vi "UI-产品孔数.vi"(8 "error in (no error)":errorcluster caption="错误输入（无错误）", 11 "名称或相对路径":string="Template Program") -> (0 "error in (no error) 2":errorcluster caption="错误输入（无错误）")   [LabVIEW 2017]
uses:
  Picture/SaveButtom.ctl
  <vilib>/vision/Contour.llb/IMAQ Connect Range Setting.ctl
  <vilib>/vision/Contour.llb/IMAQ Contour Curve Extraction.ctl
  Global System.vi
  <vilib>/Utility/xml.llb/Read From XML File(string).vi
  <vilib>/Utility/xml.llb/Write to XML File(string).vi
panel:
  in  "图像获取":bool
  in  "Curve Extraction (Contour Analysis 1)":T1={"Extraction Mode"=0, "Edge Threshold"=75, "Edge Filter Size"=0, "Min Length"=25, "Search Step Size"=15, "Max Endpoint Gap"=10, "Subpixel"=TRUE} {"Extraction Mode" items=["Normal", "Uniform Regions"]; "Edge Filter Size" items=["Fine", "Normal", "Contour Tracing"]; "Max Endpoint Gap" min=0; "Search Step Size" min=1 max=255 step=1; "Min Length" min=0; "Edge Threshold" min=1 max=350 step=1}
  in  "Match Mode (Contour Analysis 1)":T2
  in  "Template File Path (Contour Analysis 1)":path=path "C:/Users/hedongpo/Desktop/吕亚/Temp3.png"
  in  "Kernel Width (Contour Analysis 1)":u32=5
  in  "Smoothing Kernel (Contour Analysis 1)":u32
  in  "Curve Extraction 2 (Contour Analysis 1)":T1={"Extraction Mode"=0, "Edge Threshold"=75, "Edge Filter Size"=0, "Min Length"=25, "Search Step Size"=15, "Max Endpoint Gap"=10, "Subpixel"=TRUE} {"Extraction Mode" items=["Normal", "Uniform Regions"]; "Edge Filter Size" items=["Fine", "Normal", "Contour Tracing"]; "Max Endpoint Gap" min=0; "Search Step Size" min=1 max=255 step=1; "Min Length" min=0; "Edge Threshold" min=1 max=350 step=1}
  in  "Curve Connection (Contour Analysis 1)":T3[](array[typedef])=[{"Match Constraints"=0, "Min"=1.0, "Max"=12.0}] {"Max" format="%.2f"; "Min" format="%.2f"; "Match Constraints" items=["Distance (pixel)", "Angle Difference (degrees)", "Connectivity Distance (pixel)", "Gradient Difference (degrees)"]}
  in  "Contour Selection (Contour Analysis 1)":T4(ring)
  in  "Search Direction (Contour Analysis 1)":T5(ring)=enum."Annulus Outer To Inner"
  in  "刷新":bool
  in  "测试按钮":bool
  in  "保存按钮":bool
  in  "Main":enum32{"主参数", "显示", "孔数参数设置", "测试效果"}(tab)
  in  "ParamsUI":T6 caption="参数界面" {"Exposure Values" scale=0.0..200000.0}
  out "模板制作":T7(plugin-control)
  in  "抓边参数":T8={"二值化参数"={"Lower value"=104.0, "Upper value"=255.0}, "Selection Values"=[{"Measurement Parameter"=35, "Range Lower Value"=1949.8375244140625, "Range Upper Value"=6069341.0, "Range"=FALSE, "Measurement Type"=FALSE}], "Selection Values2"=[{"Measurement Parameter"=19, "Range Lower Value"=98.74, "Range Upper Value"=135.92, "Range"=FALSE, "Measurement Type"=FALSE}]} caption="参数界面" {"Selection Values2"."Measurement Parameter" items=["Center of Mass X", "Center of Mass Y", "First Pixel X", "First Pixel Y", "Bounding Rect Left", "Bounding Rect Top", "Bounding Rect Right", "Bounding Rect Bottom", "Max Feret Diameter Start X", "Max Feret Diameter Start Y", "Max Feret Diameter End X", "Max Feret Diameter End Y", "Max Horiz. Segment Length Left", "Max Horiz. Segment Length Right", "Max Horiz. Segment Length Row", "-", "Bounding Rect Width", "Bounding Rect Height", "Bounding Rect Diagonal", "Perimeter", "Convex Hull Perimeter", "Holes' Perimeter", "Max Feret Diameter", "Equivalent Ellipse Major Axis", "Equivalent Ellipse Minor Axis", "Equivalent Ellipse Minor Axis (Feret)", "Equivalent Rect Long Side", "Equivalent Rect Short Side", "Equivalent Rect Diagonal", "Equivalent Rect Short Side (Feret)", "Average Horiz. Segment Length", "Average Vert. Segment Length", "Hydraulic Radius", "Waddel Disk Diameter", "-", "Area", "Holes' Area", "Particle & Holes' Area", "Convex Hull Area", "Image Area", "-", "Number of Holes", "Number of Horiz. Segments", "Number of Vert. Segments", "-", "Orientation", "Max Feret Diameter Orientation", "-", "% Area/Image Area", "% Area/(Particle & Holes' Area)", "Ratio of Equivalent Ellipse Axes", "Ratio of Equivalent Rect Sides", "-", "Elongation Factor", "Compactness Factor", "Heywood Circularity Factor", "Type Factor", "-", "Sum X", "Sum Y", "Sum XX", "Sum XY", "Sum YY", "Sum XXX", "Sum XXY", "Sum XYY", "Sum YYY", "-", "Moment of Inertia XX", "Moment of Inertia XY", "Moment of Inertia YY", "Moment of Inertia XXX", "Moment of Inertia XXY", "Moment of Inertia XYY", "Moment of Inertia YYY", "Norm. Moment of Inertia XX", "Norm. Moment of Inertia XY", "Norm. Moment of Inertia YY", "Norm. Moment of Inertia XXX", "Norm. Moment of Inertia XXY", "Norm. Moment of Inertia XYY", "Norm. Moment of Inertia YYY", "Hu Moment 1", "Hu Moment 2", "Hu Moment 3", "Hu Moment 4", "Hu Moment 5", "Hu Moment 6", "Hu Moment 7"]; "Selection Values"."Measurement Parameter" items=["Center of Mass X", "Center of Mass Y", "First Pixel X", "First Pixel Y", "Bounding Rect Left", "Bounding Rect Top", "Bounding Rect Right", "Bounding Rect Bottom", "Max Feret Diameter Start X", "Max Feret Diameter Start Y", "Max Feret Diameter End X", "Max Feret Diameter End Y", "Max Horiz. Segment Length Left", "Max Horiz. Segment Length Right", "Max Horiz. Segment Length Row", "-", "Bounding Rect Width", "Bounding Rect Height", "Bounding Rect Diagonal", "Perimeter", "Convex Hull Perimeter", "Holes' Perimeter", "Max Feret Diameter", "Equivalent Ellipse Major Axis", "Equivalent Ellipse Minor Axis", "Equivalent Ellipse Minor Axis (Feret)", "Equivalent Rect Long Side", "Equivalent Rect Short Side", "Equivalent Rect Diagonal", "Equivalent Rect Short Side (Feret)", "Average Horiz. Segment Length", "Average Vert. Segment Length", "Hydraulic Radius", "Waddel Disk Diameter", "-", "Area", "Holes' Area", "Particle & Holes' Area", "Convex Hull Area", "Image Area", "-", "Number of Holes", "Number of Horiz. Segments", "Number of Vert. Segments", "-", "Orientation", "Max Feret Diameter Orientation", "-", "% Area/Image Area", "% Area/(Particle & Holes' Area)", "Ratio of Equivalent Ellipse Axes", "Ratio of Equivalent Rect Sides", "-", "Elongation Factor", "Compactness Factor", "Heywood Circularity Factor", "Type Factor", "-", "Sum X", "Sum Y", "Sum XX", "Sum XY", "Sum YY", "Sum XXX", "Sum XXY", "Sum XYY", "Sum YYY", "-", "Moment of Inertia XX", "Moment of Inertia XY", "Moment of Inertia YY", "Moment of Inertia XXX", "Moment of Inertia XXY", "Moment of Inertia XYY", "Moment of Inertia YYY", "Norm. Moment of Inertia XX", "Norm. Moment of Inertia XY", "Norm. Moment of Inertia YY", "Norm. Moment of Inertia XXX", "Norm. Moment of Inertia XXY", "Norm. Moment of Inertia XYY", "Norm. Moment of Inertia YYY", "Hu Moment 1", "Hu Moment 2", "Hu Moment 3", "Hu Moment 4", "Hu Moment 5", "Hu Moment 6", "Hu Moment 7"]; "Selection Values"."Range Upper Value" format="%#_9f"}
  in  "测试结果":string[][](table)=[["", ""]]
  out "原始图像":T7(plugin-control)
  out "处理后图像":T7(plugin-control)
  out "路径输出":path
  out "添加的路径":path
  in  "Vision Paramter Save Buttom":T9
  out "system time":string
  in  "取消按钮":bool
  # "Range"
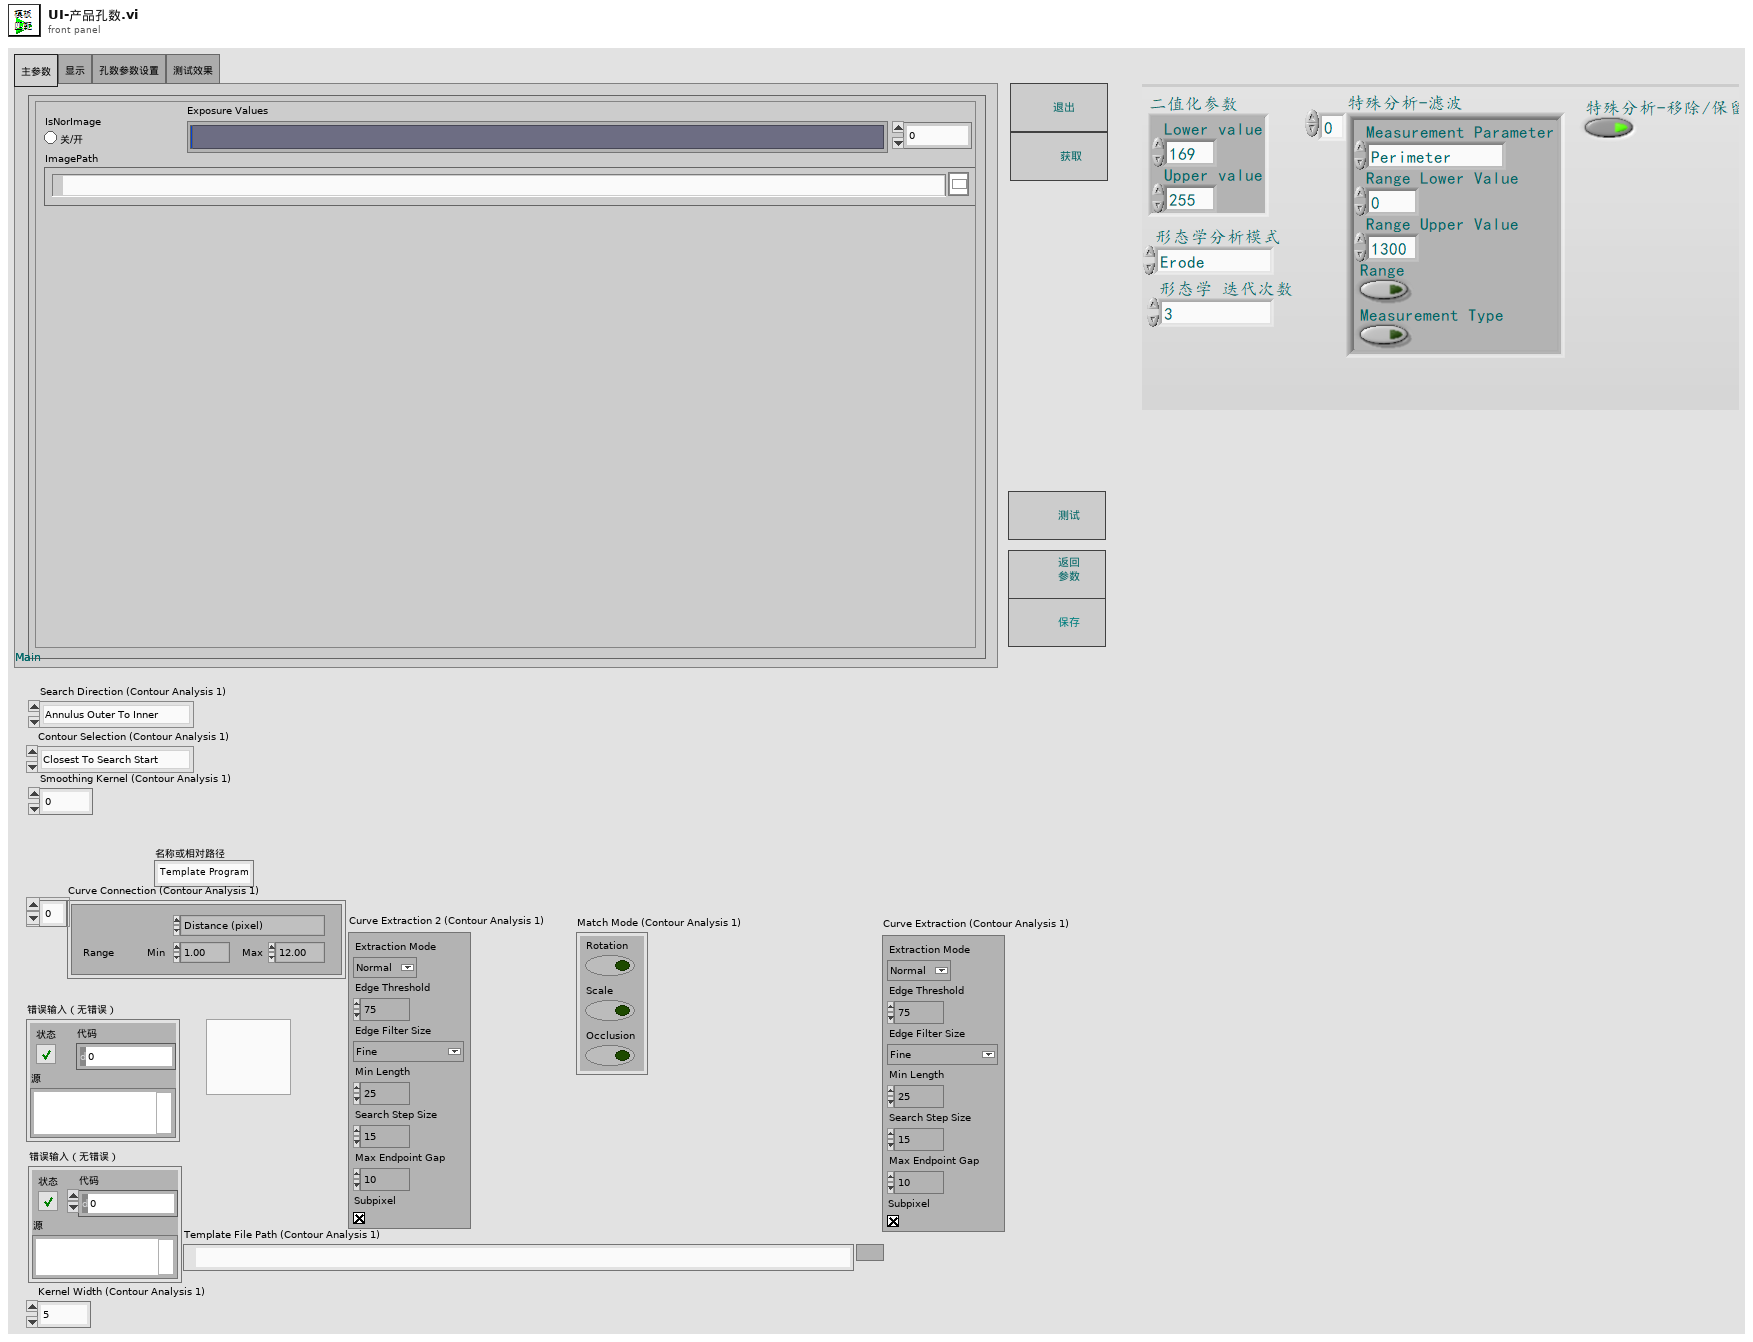
[diagram p1: front panel]
types:
  T1 = typedef "IMAQ Contour Curve Extraction.ctl" = cluster{"Extraction Mode":u32, "Edge Threshold":i32, "Edge Filter Size":u32, "Min Length":i32, "Search Step Size":i32, "Max Endpoint Gap":i32, "Subpixel":bool}
  T2 = cluster{"Rotation":bool, "Scale":bool, "Occlusion":bool}
  T3 = typedef "IMAQ Connect Range Setting.ctl" = cluster{"Match Constraints":u32, "Min":dbl, "Max":dbl}
  T4 = enum16{"Closest To Search Start", "Maximum Length", "Strongest Mean Gradient Change"}
  T5 = enum16{"Rect Left To Right", "Rect Right To Left", "Rect Top To Bottom", "Rect Bottom To Top", "Annulus Inner To Outer", "Annulus Outer To Inner", "Annulus Start Angle To End Angle", "Annulus End Angle To Start Angle"}
  T6 = cluster{"IsNorImage":bool, "Exposure Values":u32, "ImagePath":path}
  T7 = typedef "IMAQ Image.ctl" = refnum<image>
  T8 = cluster{"二值化参数":cluster{"Lower value":sgl, "Upper value":sgl}, "Selection Values":cluster{"Measurement Parameter":i32, "Range Lower Value":dbl, "Range Upper Value":dbl, "Range":bool, "Measurement Type":bool}[], "Selection Values2":cluster{"Measurement Parameter":i32, "Range Lower Value":dbl, "Range Upper Value":dbl, "Range":bool, "Measurement Type":bool}[]}
  T9 = typedef "SaveButtom.ctl" = bool
  T10 = cluster{"index":i32, "this vi":refnum<vi>, "error out":errorcluster}
  T11 = cluster{"master data":string, "priority":u16, "secondary data":string[]}
  T12 = cluster{"case name":string[], "queue array":refnum<queue>[]}
  T13 = typedef "Image Type" = u32
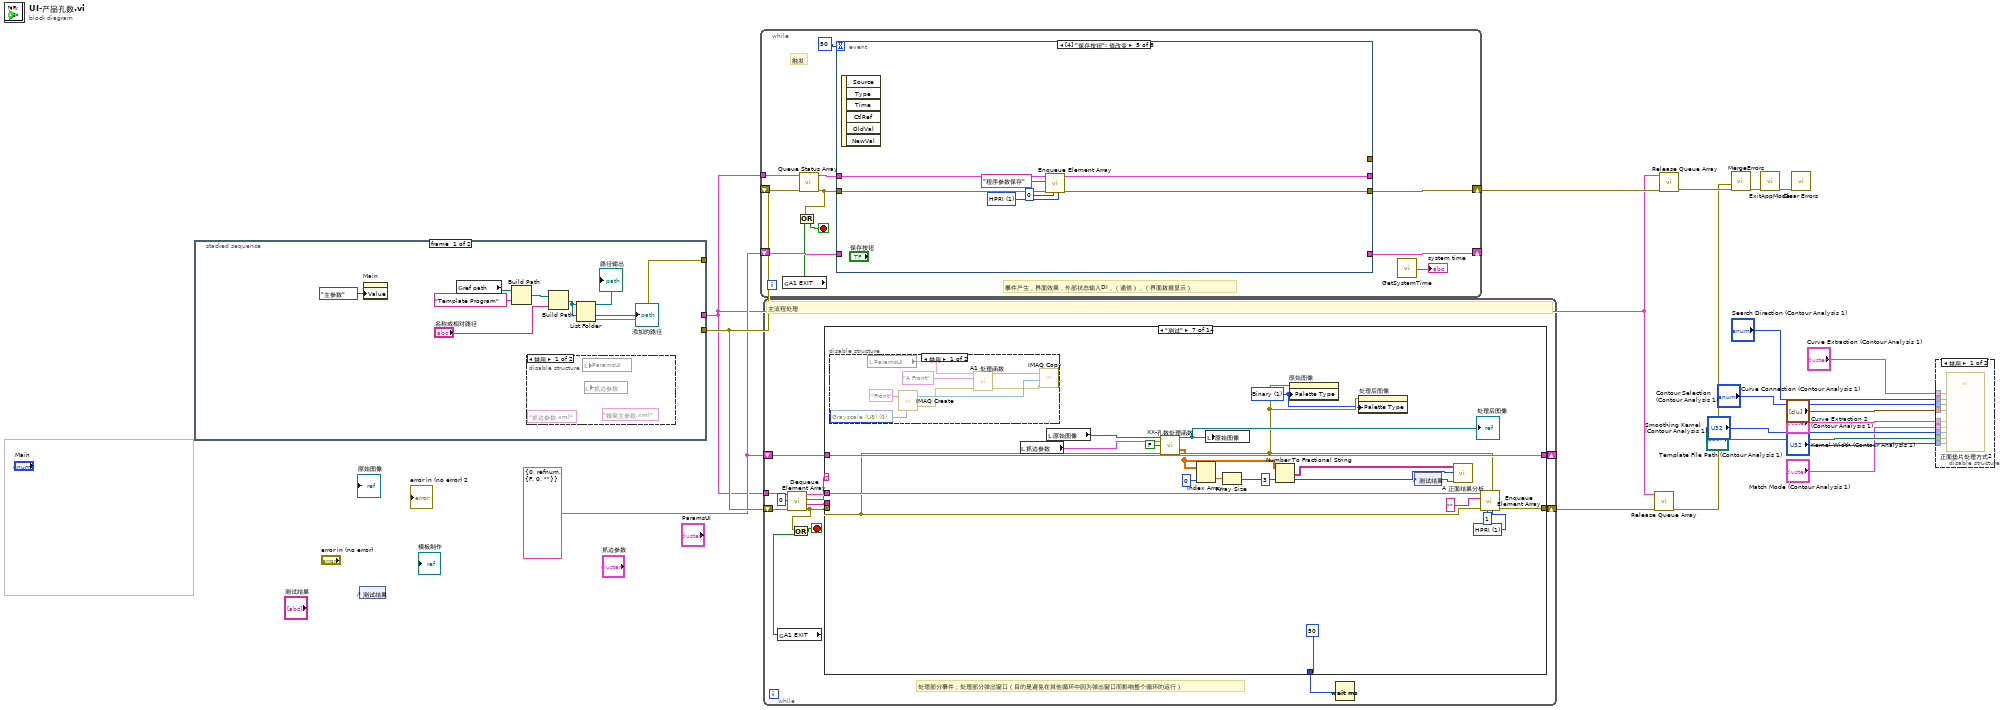
[diagram p0: block diagram]
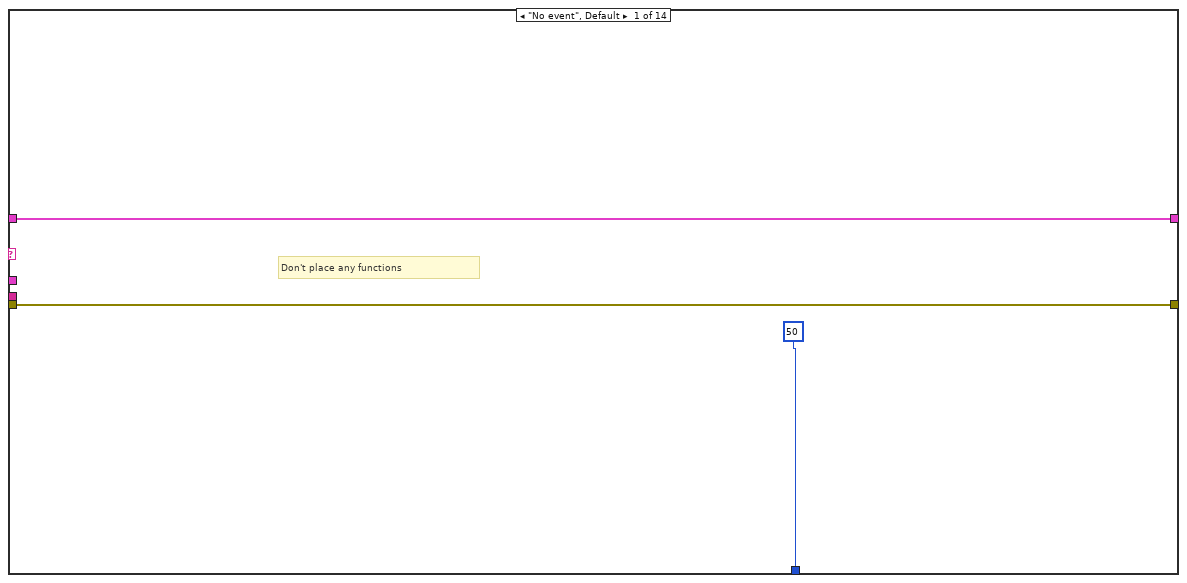
[diagram p3: hidden frame]
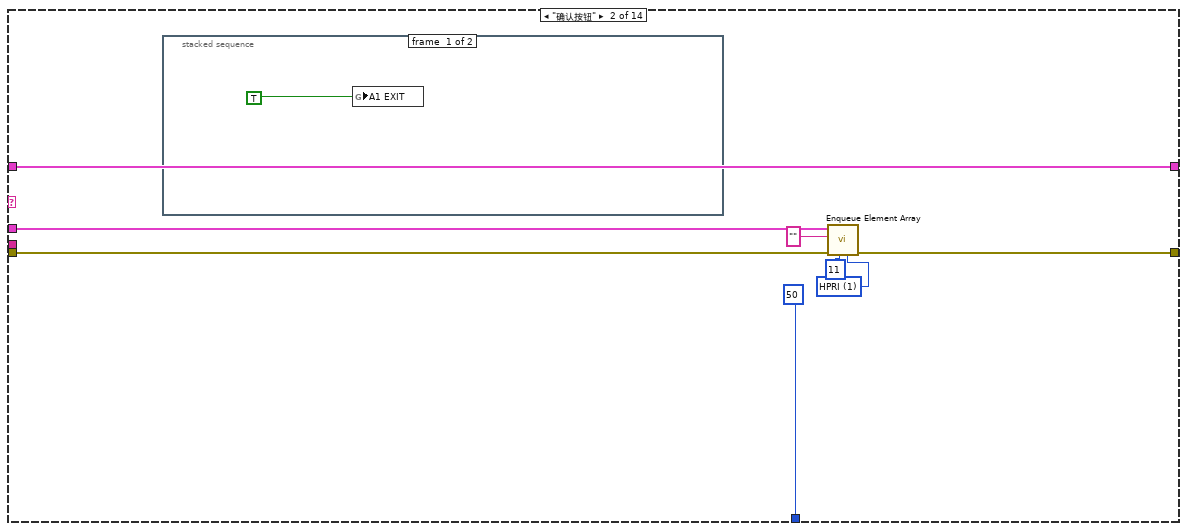
[diagram p4: hidden frame]
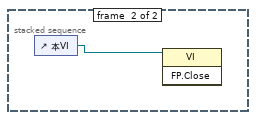
[diagram p5: hidden frame]
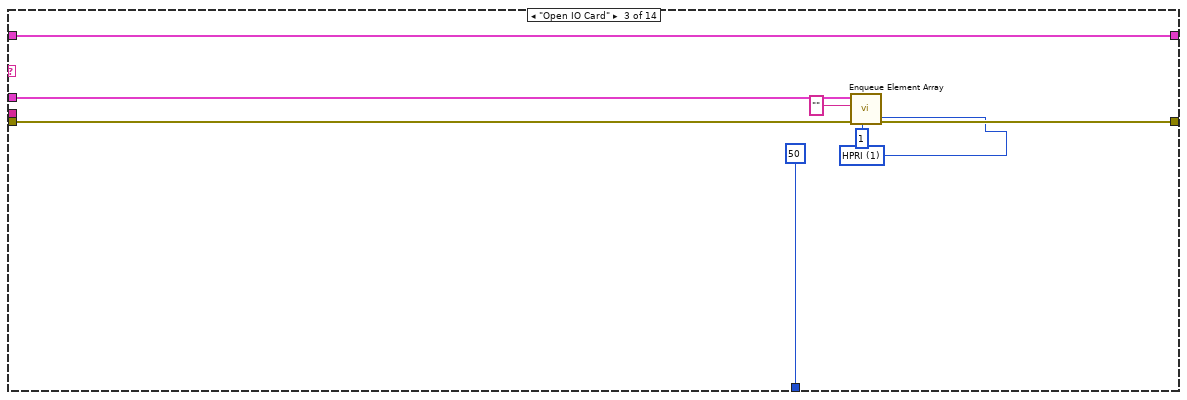
[diagram p6: hidden frame]
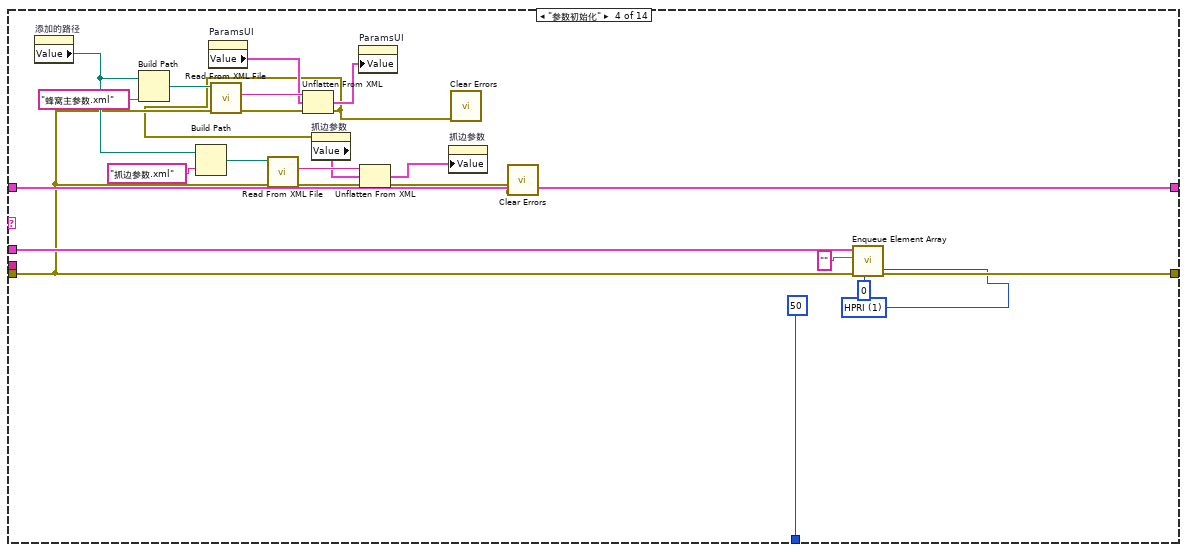
[diagram p7: hidden frame]
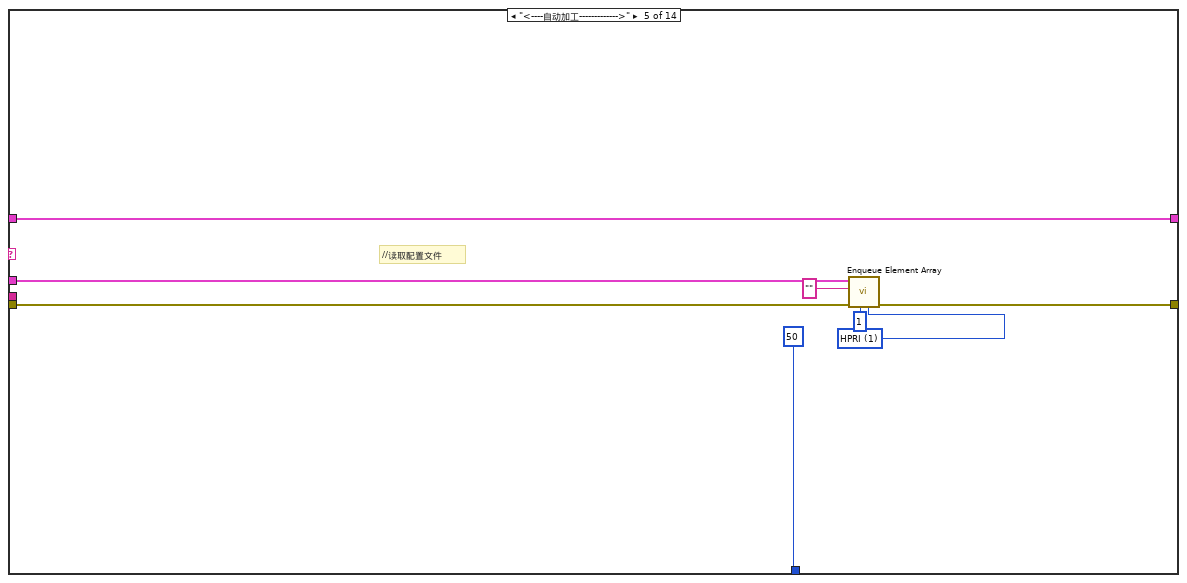
[diagram p8: hidden frame]
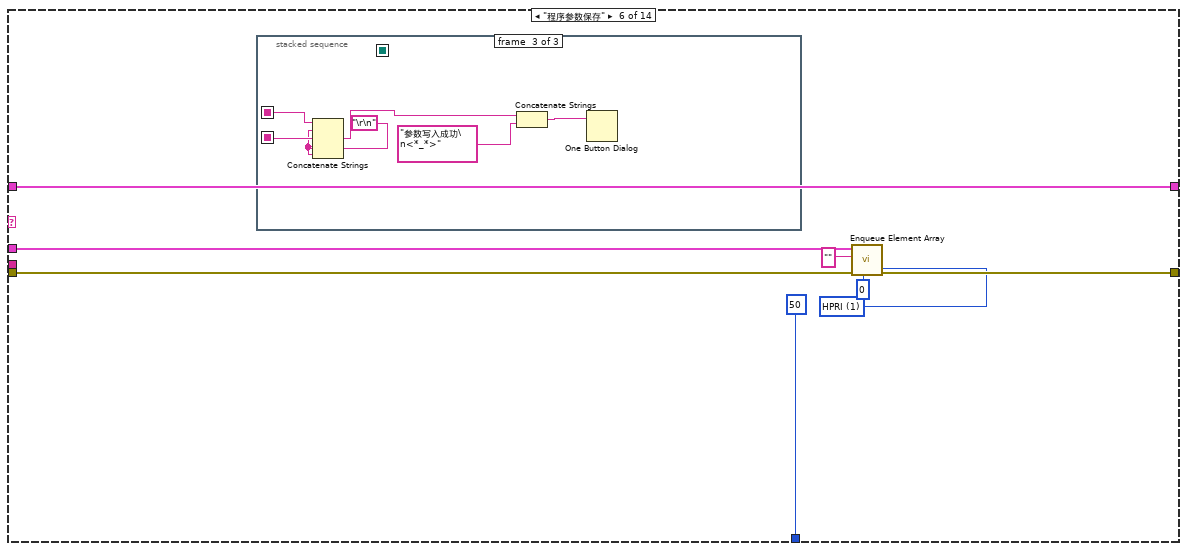
[diagram p9: hidden frame]
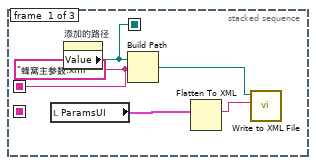
[diagram p10: hidden frame]
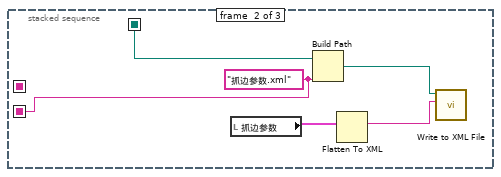
[diagram p11: hidden frame]
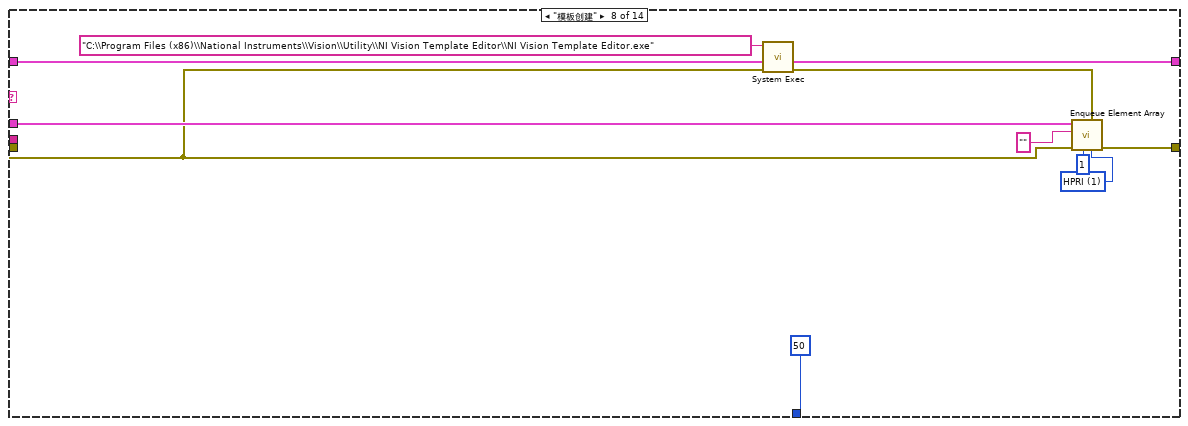
[diagram p13: hidden frame]
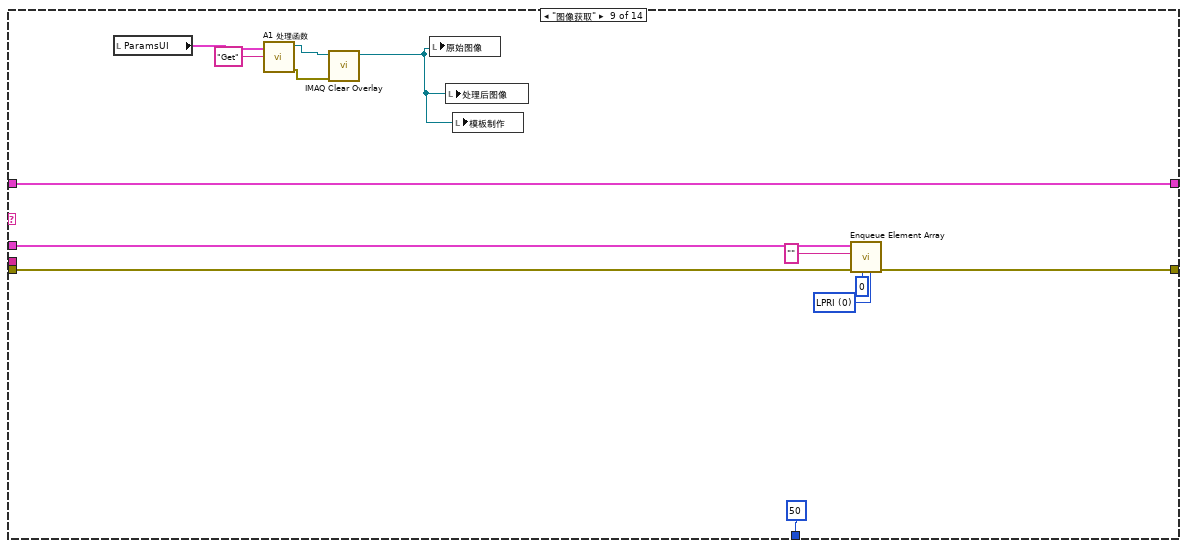
[diagram p14: hidden frame]
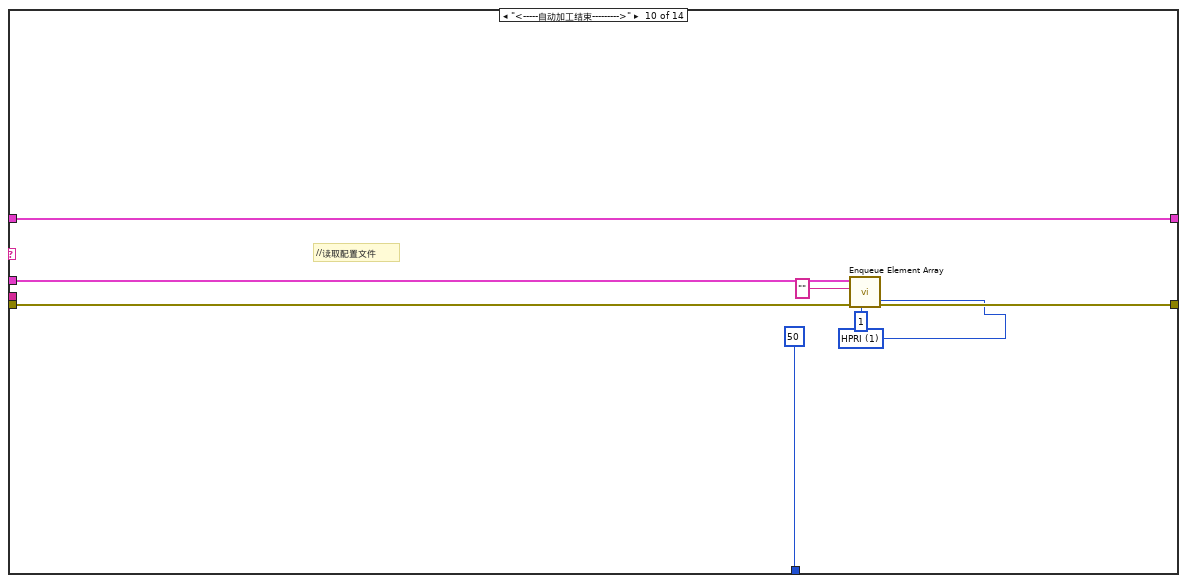
[diagram p15: hidden frame]
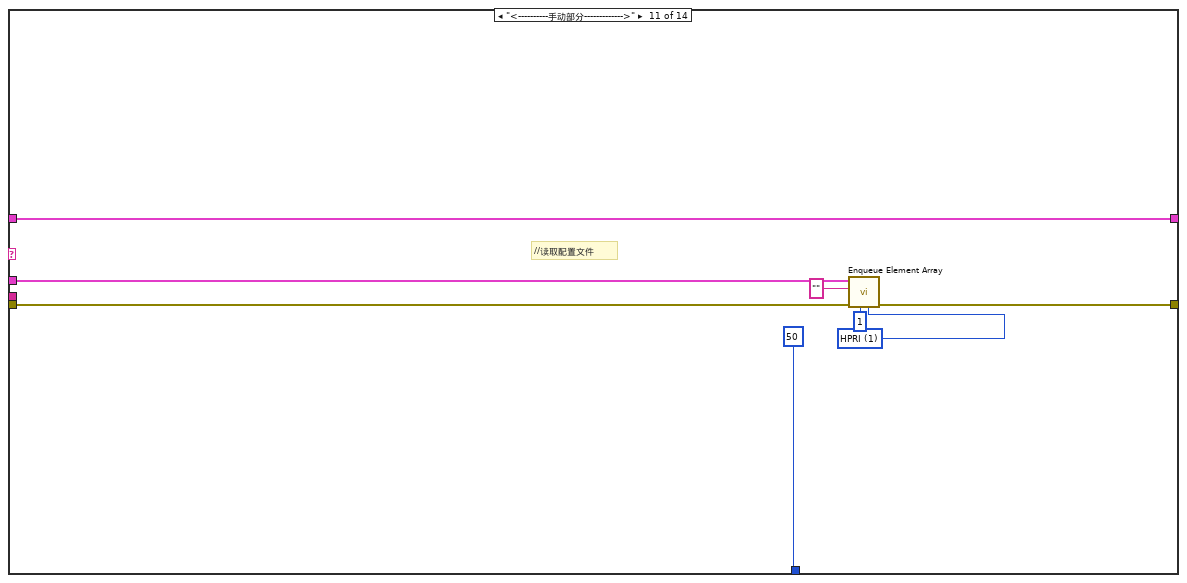
[diagram p16: hidden frame]
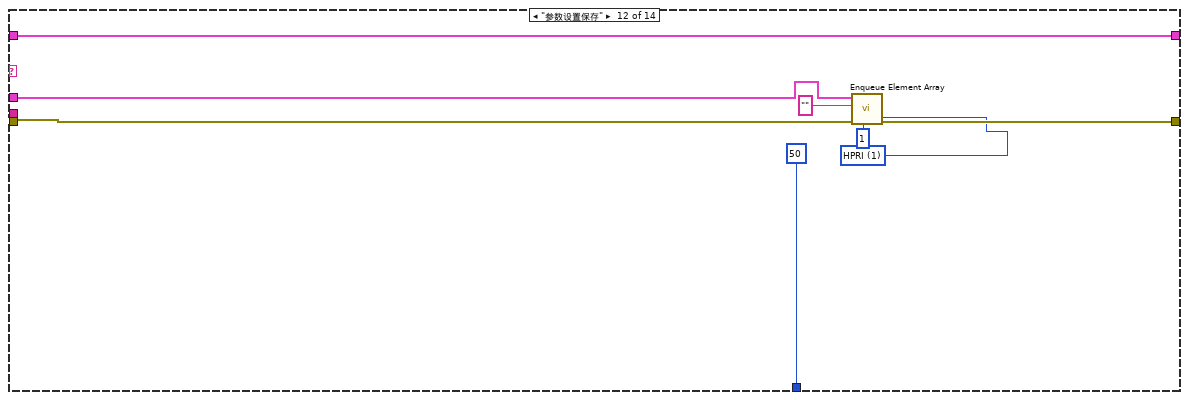
[diagram p17: hidden frame]
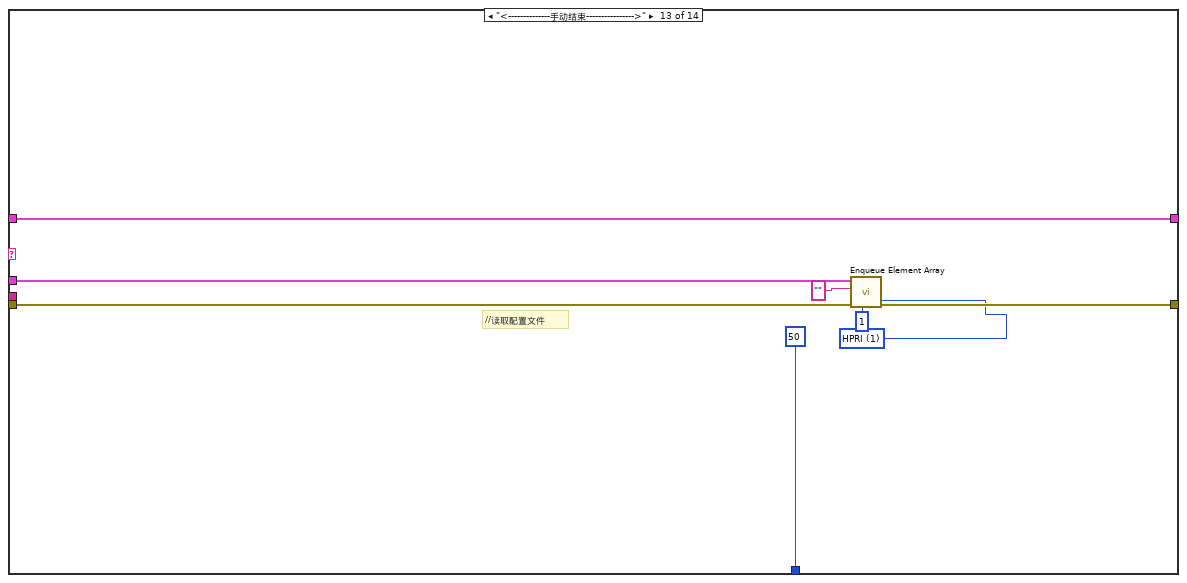
[diagram p18: hidden frame]
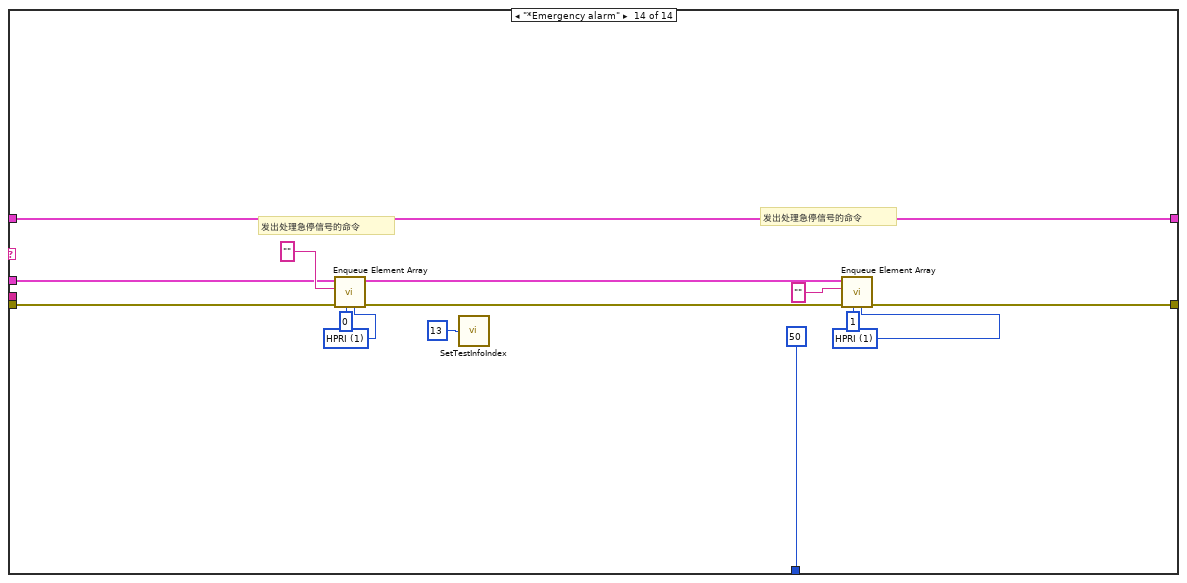
[diagram p19: hidden frame]
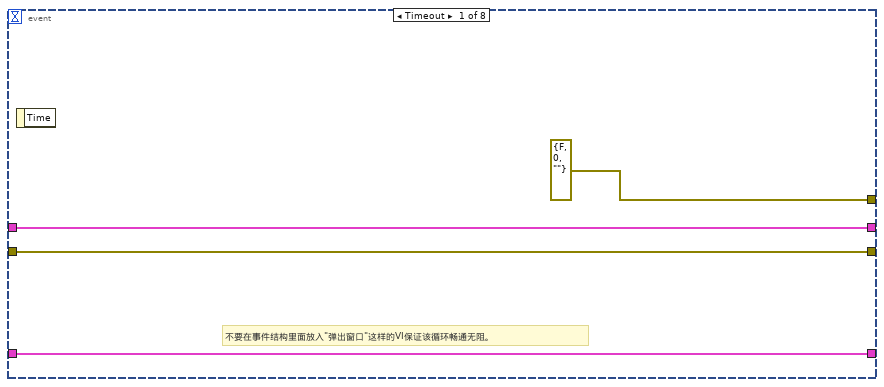
[diagram p20: hidden frame]
diagram:
  w13 = T10 {"index"=0, "this vi"=refnum, "error out"={"status"=FALSE, "code"=0, "source"=""}} ("parameter buffer")
  n1 = stacked-sequence {
    tunnel: [w24 _] -> _
    tunnel: [_ w28] -> w14
    tunnel: [_ w27] -> w10
    frame #0 {
      n2 = property on="Main" class="TabCtl (严格)"("Value"=enum32{"主参数", "显示", "孔数参数设置", "测试效果"}."主参数" ("Main")) -> ()  [unwired: 2 in, 2 out]
      n3 = global read "Global System.vi" "ref path"() -> (w22:path)
      n4 = Build Path(base path=w22, name or relative path="Template Program" ("名称或相对路径")) -> (appended path=w20:path)
      n5 = disable-structure shown="禁用" {
        frame Disabled {
          (unwired) "抓边参数.xml" ("名称或相对路径")
          (unwired) "蜂窝主参数.xml" ("名称或相对路径")
          n6 = local read "ParamsUI"() -> ()  [unwired: 1 in]
          n7 = local read "抓边参数"() -> ()  [unwired: 1 in]
        }
        frame Enabled {
        }
      }
      n8 = Build Path(base path=w20, name or relative path="名称或相对路径") -> (appended path=w26:path)
      "添加的路径" <- w26
      n9 = List Folder(path=w26) -> (path out=→"路径输出":path, error out=w24:errorcluster)  [unwired: 3 in, 2 out]
    }
    frame #1 {
      w36 = string[] ["comm queue1", "data queue 11", "data queue 12", "data queue 13", "data queue 14"]  # queue name
      w37 = 4  # queue num
      w38 = T11 {"master data"="", "priority"=0, "secondary data"=[]}  # element data type
      n10 = call "Obtain Queue Array.vi"("queue name"=w36, "element data type"=w38, "queue num"=w37) -> ("error out"=w32:errorcluster, "queue out"=w33:T12)  [unwired: 2 in, 1 out]
      n11 = call "Enqueue Element Array.vi"("queue index"=0, "error in"=w32, "master data"="参数初始化", "queue in"=w33) -> ("error out"=w31:errorcluster, "queue out"=w30:T12)  [unwired: 6 in]
      n12 = disable-structure shown="启用" {
        disable-tunnel: w31 -> [w44 w45]
        disable-tunnel: w30 -> [w43 w46]
        disable-tunnel: "Loading Variable" ("master data") -> [w42 _]
        disable-tunnel: [w40 w45] -> w28
        disable-tunnel: [w39 w46] -> w27
        frame Disabled {
          n13 = call "Enqueue Element Array.vi"("queue index"=12, "error in"=w44, "master data"=w42, "queue in"=w43) -> ("error out"=w40:errorcluster, "queue out"=w39:T12)  [unwired: 6 in]
        }
        frame Enabled {
        }
      }
    }
  }
  n14 = control-ref of="测试结果"() -> ()  [unwired: 1 out]
  n15 = while {
    shift-right: [w50] -> w15
    shift-left: w14 -> [w54]
    shift-right: [w52] -> _
    shift-left: w13 -> [w53]
    tunnel: w10 -> [w56]
    stop <- w47 stop-if-true
    # "触发"
    # "事件产生，界面效果，外部状态输入DI，（通信），（界面数据显示）"
    n16 = global read "Global System.vi" "A1 EXIT"() -> (w48:bool)
    n17 = call "Queue Status Array.vi"("error in (no error)"=w54, "queue in"=w56) -> ("error out"=w49:errorcluster, "queue out"=w51:T12)  [unwired: 4 in]
    n18 = Or(x=w49, y=w48) -> (x .or. y?=w47:bool)
    n19 = event shown="[4] \"保存按钮\": 值改变" {
      selector: _ -> [_ _ _ _ _ _ _ _]
      dyn-events: _ -> [_ _ _ _ _ _ _ _]
      timeout: 50 -> [_ _ _ _ _ _ _ _]
      tunnel: w53 -> [w61 w69 _ _ _ _ _ _]
      tunnel: [w61 w69 _ _ _ _ _ _] -> w52
      tunnel: [errorcluster {"status"=FALSE, "code"=0, "source"=""} ("error out") _ _ _ _ _ _ _] -> _
      tunnel: w51 -> [w59 w68 w74 w81 w88 w96 w104 w112]
      tunnel: w49 -> [w58 w67 w73 w80 w87 w95 w103 w111]
      tunnel: [w58 w66 w71 w78 w85 w93 w101 w109] -> w50
      tunnel: [w59 w65 w72 w79 w86 w94 w102 w110] -> _
      event Timeout {
        # "不要在事件结构里面放入\"弹出窗口\"这样的VI保证该循环畅通无阻。"
        n20 = event-data() -> ()  [unwired: 1 in, 1 out]
      }
      event Panel Close? {
        w63 = u16 1 items=["HPRI"=1, "LPRI"=0] ("priority")
        n21 = event-data() -> ()  [unwired: 1 in, 4 out]
        n22 = call "Enqueue Element Array.vi"("priority"=w63, "queue index"=0, "error in"=w67, "master data"="*Exit application", "queue in"=w68) -> ("error out"=w66:errorcluster, "queue out"=w65:T12)  [unwired: 5 in]
        n23 = event-data("Discard?"=TRUE) -> ()  [unwired: 1 in, 1 out]
      }
      event Value Change {
        w76 = u16 1 items=["HPRI"=1, "LPRI"=0] ("priority")
        n24 = event-data() -> ()  [unwired: 1 in, 6 out]
        n25 = call "Enqueue Element Array.vi"("priority"=w76, "queue index"=0, "error in"=w73, "master data"="Vision Paramter Save", "queue in"=w74) -> ("error out"=w71:errorcluster, "queue out"=w72:T12)  [unwired: 5 in]
      }
      event "取消按钮": Value Change {
        w83 = u16 1 items=["HPRI"=1, "LPRI"=0] ("priority")
        n26 = event-data() -> ()  [unwired: 1 in, 6 out]
        n27 = call "Enqueue Element Array.vi"("priority"=w83, "queue index"=0, "error in"=w80, "master data"="确认按钮", "queue in"=w81) -> ("error out"=w78:errorcluster, "queue out"=w79:T12)  [unwired: 5 in]
      }
      event "保存按钮": Value Change {
        w90 = u16 1 items=["HPRI"=1, "LPRI"=0] ("priority")
        n28 = event-data() -> ()  [unwired: 1 in, 6 out]
        n29 = call "Enqueue Element Array.vi"("priority"=w90, "queue index"=0, "error in"=w87, "master data"="程序参数保存", "queue in"=w88) -> ("error out"=w85:errorcluster, "queue out"=w86:T12)  [unwired: 5 in]
      }
      event "测试按钮": Value Change {
        (unwired) "模板匹配抓边测试"
        w98 = u16 1 items=["HPRI"=1, "LPRI"=0] ("priority")
        n30 = event-data() -> ()  [unwired: 1 in, 6 out]
        n31 = property on="Main" class="TabCtl (严格)"("Value"=enum32{"主参数", "显示", "孔数参数设置", "测试效果"}."测试效果" ("Main")) -> ()  [unwired: 2 in, 2 out]
        n32 = call "Enqueue Element Array.vi"("priority"=w98, "queue index"=0, "error in"=w95, "master data"="测试", "queue in"=w96) -> ("error out"=w93:errorcluster, "queue out"=w94:T12)  [unwired: 5 in]
      }
      event "图像获取": Value Change {
        w106 = u16 1 items=["HPRI"=1, "LPRI"=0] ("priority")
        n33 = event-data() -> ()  [unwired: 1 in, 6 out]
        n34 = property on="Main" class="TabCtl (严格)"("Value"=enum32{"主参数", "显示", "孔数参数设置", "测试效果"}."显示" ("Main")) -> ()  [unwired: 2 in, 2 out]
        n35 = call "Enqueue Element Array.vi"("priority"=w106, "queue index"=0, "error in"=w103, "master data"="图像获取", "queue in"=w104) -> ("error out"=w101:errorcluster, "queue out"=w102:T12)  [unwired: 5 in]
      }
      event "刷新": Value Change {
        n36 = event-data() -> ()  [unwired: 1 in, 6 out]
        n37 = disable-structure shown="禁用" {
          disable-tunnel: w112 -> [w116 _]
          disable-tunnel: w111 -> [w115 _]
          disable-tunnel: [w114 _] -> w110
          disable-tunnel: [w113 _] -> w109
          frame Disabled {
            w118 = u16 1 items=["HPRI"=1, "LPRI"=0] ("priority")
            # "刷新"
            n38 = call "Enqueue Element Array.vi"("priority"=w118, "queue index"=0, "error in"=w115, "master data"="刷新", "queue in"=w116) -> ("error out"=w113:errorcluster, "queue out"=w114:T12)  [unwired: 5 in]
          }
          frame Enabled {
          }
        }
        n39 = property on="Main" class="TabCtl (严格)"("Value"=enum32{"主参数", "显示", "孔数参数设置", "测试效果"}."主参数" ("Main")) -> ()  [unwired: 2 in, 2 out]
      }
    }
    n40 = call "GetSystemTime.vi"() -> ("date/time string"=→"system time":string)  [unwired: 7 in]
  }
  n41 = while {
    shift-right: [w132] -> w12
    shift-left: w14 -> [w123]
    shift-right: [w129] -> _
    shift-left: w13 -> [w130]
    tunnel: w10 -> [w125]
    stop <- w120 stop-if-true
    # "处理部分事件；处理部分弹出窗口（目的是避免在其他循环中因为弹出窗口而影响整个循环的运行）"
    # "主流程处理"
    n42 = global read "Global System.vi" "A1 EXIT"() -> (w121:bool)
    n43 = call "Dequeue Element Array.vi"("queue in"=w125, "queue index"=0, "error in"=w123) -> ("queue out"=w128:T12, "master data"=w127:string, "secondary data"=w126:string[], "error out"=w122:errorcluster)  [unwired: 2 in, 1 out]
    n44 = Or(x=w122, y=w121) -> (x .or. y?=w120:bool)
    n45 = case shown="\"测试\"" w127 {
      tunnel: w128 -> [_ w142 w152 w175 w183 w185 w228 w246 w259 w267 w275 w283 w291 w297]
      tunnel: w122 -> [w134 w138 w148 w157 w179 w189 w219 w240 w253 w263 w271 w279 w287 w294]
      tunnel: [w134 w141 w151 w174 w182 w191 w227 w245 w258 w266 w274 w282 w290 w305] -> w132
      tunnel: [50 50 50 50 50 50 50 50 50 50 50 50 50 50] -> w131
      tunnel: w130 -> [w135 w139 w149 w170 w180 w186 w226 w241 w254 w264 w272 w280 w288 w303]
      tunnel: [w135 w139 w149 w170 w180 w186 w226 w241 w254 w264 w272 w280 w288 w303] -> w129
      tunnel: w126 -> [_ _ _ _ _ _ _ _ _ _ _ _ _ _]
      frame "No event", Default {
        # "Don't place any functions"
      }
      frame "确认按钮" {
        w136 = u16 1 items=["HPRI"=1, "LPRI"=0] ("priority")
        n46 = stacked-sequence {
          frame #0 {
            n47 = global write "Global System.vi" "A1 EXIT"(TRUE ("EXIT")) -> ()
          }
          frame #1 {
            n48 = control-ref of="本VI"() -> (w145:refnum<vi>)
            n49 = invoke class="VI" method="FP.Close"(reference=w145) -> ()  [unwired: 2 in, 3 out]
          }
        }
        n50 = call "Enqueue Element Array.vi"("priority"=w136, "queue index"=11, "error in"=w138, "master data"="" ("Element 1"), "queue in"=w142) -> ("error out"=w141:errorcluster)  [unwired: 5 in, 1 out]
      }
      frame "Open IO Card" {
        w146 = u16 1 items=["HPRI"=1, "LPRI"=0] ("priority")
        n51 = call "Enqueue Element Array.vi"("priority"=w146, "queue index"=1, "error in"=w148, "master data"="" ("Element 1"), "queue in"=w152) -> ("error out"=w151:errorcluster)  [unwired: 5 in, 1 out]
      }
      frame "参数初始化" {
        w171 = u16 1 items=["HPRI"=1, "LPRI"=0] ("priority")
        n52 = property on="添加的路径" class="Path"() -> ("Value"=w159:path)  [unwired: 2 in, 2 out]
        n53 = Build Path(base path=w159, name or relative path="蜂窝主参数.xml" ("名称或相对路径")) -> (appended path=w168:path)
        n54 = Build Path(base path=w159, name or relative path="抓边参数.xml" ("名称或相对路径")) -> (appended path=w160:path)
        n55 = property on="ParamsUI" class="Clust (严格)"() -> ("Value"=w166:T6)  [unwired: 2 in, 2 out]
        n56 = call-poly <vilib>:"Read From XML File.vi"("error in (no error)"=w157, "XML File Path"=w168) -> ("error out"=w164:errorcluster, "XML Elements"=w167:string)  [unwired: 7 in, 1 out]
        n57 = call-poly <vilib>:"Read From XML File.vi"("error in (no error)"=w157, "XML File Path"=w160) -> ("error out"=w162:errorcluster, "XML Elements"=w161:string)  [unwired: 7 in, 1 out]
        n58 = Unflatten From XML(xml string=w167, type=w166, error in (no error)=w164) -> (value=w165:T6, error out=w156:errorcluster)
        n59 = property on="抓边参数" class="Clust (严格)"(error in=w156) -> ("Value"=w155:T8)  [unwired: 1 in, 2 out]
        n60 = property on="ParamsUI" class="Clust (严格)"("Value"=w165) -> ()  [unwired: 2 in, 2 out]
        n61 = Unflatten From XML(xml string=w161, type=w155, error in (no error)=w162) -> (value=w154:T8, error out=w163:errorcluster)
        n62 = property on="抓边参数" class="Clust (严格)"("Value"=w154) -> ()  [unwired: 2 in, 2 out]
        n63 = call <vilib>:"Clear Errors.vi"("error in (no error)"=w156) -> ()  [unwired: 5 in, 2 out]
        n64 = call <vilib>:"Clear Errors.vi"("error in (no error)"=w163) -> ()  [unwired: 5 in, 2 out]
        n65 = call "Enqueue Element Array.vi"("priority"=w171, "queue index"=0, "error in"=w157, "master data"="" ("Element 1"), "queue in"=w175) -> ("error out"=w174:errorcluster)  [unwired: 5 in, 1 out]
      }
      frame "<----自动加工------------->" {
        w177 = u16 1 items=["HPRI"=1, "LPRI"=0] ("priority")
        # "//读取配置文件"
        n66 = call "Enqueue Element Array.vi"("priority"=w177, "queue index"=1, "error in"=w179, "master data"="" ("Element 1"), "queue in"=w183) -> ("error out"=w182:errorcluster)  [unwired: 5 in, 1 out]
      }
      frame "程序参数保存" {
        w187 = u16 1 items=["HPRI"=1, "LPRI"=0] ("priority")
        n67 = stacked-sequence {
          seq-local: [w195 _ _] -> [_ _ w206]
          seq-local: [_ w201 _] -> [_ _ w205]
          seq-local: [w194 _ _] -> [_ w200 _]
          frame #0 {
            w195 = "蜂窝主参数.xml" ("名称或相对路径")
            n68 = local read "ParamsUI"() -> (w193:T6)
            n69 = property on="添加的路径" class="Path"() -> ("Value"=w194:path)  [unwired: 2 in, 2 out]
            n70 = Build Path(base path=w194, name or relative path=w195) -> (appended path=w196:path)
            n71 = Flatten To XML(anything=w193) -> (xml string=w197:string)
            n72 = call-poly <vilib>:"Write to XML File.vi"("XML Input"=w197, "XML File Path"=w196) -> ()  [unwired: 7 in, 3 out]
          }
          frame #1 {
            w201 = "抓边参数.xml" ("名称或相对路径")
            n73 = local read "抓边参数"() -> (w198:T8)
            n74 = Build Path(base path=w200, name or relative path=w201) -> (appended path=w202:path)
            n75 = Flatten To XML(anything=w198) -> (xml string=w199:string)
            n76 = call-poly <vilib>:"Write to XML File.vi"("XML Input"=w199, "XML File Path"=w202) -> ()  [unwired: 7 in, 3 out]
          }
          frame #2 {
            w203 = "\r\n"
            n77 = Concatenate Strings(w206, w203, w205, w203, w203) -> (w204:string)
            n78 = Concatenate Strings(w204, "参数写入成功\n<*_*>" ("消息")) -> (w207:string)
            n79 = One Button Dialog(message=w207) -> ()  [unwired: 1 in, 1 out]
          }
        }
        n80 = call "Enqueue Element Array.vi"("priority"=w187, "queue index"=0, "error in"=w189, "master data"="" ("Element 1"), "queue in"=w185) -> ("error out"=w191:errorcluster)  [unwired: 5 in, 1 out]
      }
      frame "测试" {
        w215 = u32 1 items=["Grayscale", "Binary", "Gradient", "Rainbow", "Temperature", "User Defined", "Binary 16 Bit", "Gradient 16 Bit", "Rainbow 16 Bit", "Temperature 16 Bit", "User Defined 16 Bit"] ("Palette:Palette Type")
        w223 = u16 1 items=["HPRI"=1, "LPRI"=0] ("priority")
        n81 = disable-structure shown="禁用" {
          frame Disabled {
            w236 = T13 0 items=["Grayscale (U8)", "Grayscale (I16)", "Grayscale (SGL)", "Complex (CSG)", "RGB (U32)", "HSL (U32)", "RGB (U64)", "Grayscale (U16)"] ("Image Type")
            n82 = local read "ParamsUI"() -> (w230:T6)
            n83 = call "IMAQ Create"("Image Name"="Front", "Image Type"=w236) -> ("New Image"=w235:T7, "error out"=w233:errorcluster)  [unwired: 3 in]
            n84 = call "A1 处理函数.vi"("error in (no error)"=w233, "Image Name"="A Front", "ParamsUI"=w230) -> ("error out"=w231:errorcluster, "Image out"=w232:T7)  [unwired: 7 in]
            n85 = call "IMAQ Copy"("error in (no error)"=w231, "Image Dst"=w235, "Image Src"=w232) -> ()  [unwired: 3 in, 2 out]
          }
          frame Enabled {
          }
        }
        n86 = local read "抓边参数"() -> (w220:T8)
        n87 = local read "原始图像"() -> (w221:T7)
        n88 = call "XX-孔数处理函数.vi"("Image in"=w221, "参数输入"=w220, "图像处理开关"=FALSE, "error in"=w219) -> ("Image Out"=w217:T7, "Particle Measurements (Pixels)"=w211:dbl[][], "error out"=w216:errorcluster)  [unwired: 9 in]
        "处理后图像" <- w217
        n89 = Index Array(array=w211, index (col)=0 ("禁用的索引 (列)")) -> (element=w213:dbl[])  [unwired: 1 in]
        n90 = local write "原始图像"(w217) -> ()
        n91 = Array Size(array=w213) -> (size(s)=w212:i32)
        n92 = Number To Fractional String(number=w211, precision (6)=i16 3 ("精度(6)")) -> (F-format string=w209:string[][])  [unwired: 2 in]
        n93 = property on="原始图像" class="ImageControl"(error in=w216, "Palette Type"=w215) -> ()  [unwired: 1 in, 2 out]
        n94 = property on="处理后图像" class="ImageControl"(error in=w216, "Palette Type"=w215) -> ()  [unwired: 1 in, 2 out]
        n95 = control-ref of="测试结果"() -> (w222:refnum<vi>)
        n96 = call "A 正面结果分析.vi"("Tbl引用句柄"=w222, "列数"=w212, "距离"=w209) -> ()  [unwired: 9 in]
        n97 = call "Enqueue Element Array.vi"("priority"=w223, "device error in"=w216, "queue index"=1, "error in"=w219, "master data"="" ("Element 1"), "queue in"=w228) -> ("error out"=w227:errorcluster)  [unwired: 4 in, 1 out]
      }
      frame "模板创建" {
        w242 = u16 1 items=["HPRI"=1, "LPRI"=0] ("priority")
        n98 = call <vilib>:"System Exec.vi"("error in (no error)"=w240, "command line"="C:\\Program Files (x86)\\National Instruments\\Vision\\Utility\\NI Vision Template Editor\\NI Vision Template Editor.exe") -> ("error out"=w239:errorcluster)  [unwired: 6 in, 3 out]
        n99 = call "Enqueue Element Array.vi"("priority"=w242, "device error in"=w239, "queue index"=1, "error in"=w240, "master data"="" ("Element 1"), "queue in"=w246) -> ("error out"=w245:errorcluster)  [unwired: 4 in, 1 out]
      }
      frame "图像获取" {
        w256 = u16 0 items=["HPRI"=1, "LPRI"=0] ("priority")
        n100 = local read "ParamsUI"() -> (w251:T6)
        n101 = call "A1 处理函数.vi"("Image Name"="Get", "ParamsUI"=w251) -> ("error out"=w249:errorcluster, "Image out"=w250:T7)  [unwired: 8 in]
        n102 = call "IMAQ Clear Overlay"("error in (no error)"=w249, "Image"=w250) -> ("Image Out"=w248:T7)  [unwired: 8 in, 1 out]
        n103 = local write "原始图像"(w248) -> ()
        n104 = local write "处理后图像"(w248) -> ()
        n105 = local write "模板制作"(w248) -> ()
        n106 = call "Enqueue Element Array.vi"("priority"=w256, "queue index"=0, "error in"=w253, "master data"="", "queue in"=w259) -> ("error out"=w258:errorcluster)  [unwired: 5 in, 1 out]
      }
      frame "<-----自动加工结束--------->" {
        w261 = u16 1 items=["HPRI"=1, "LPRI"=0] ("priority")
        # "//读取配置文件"
        n107 = call "Enqueue Element Array.vi"("priority"=w261, "queue index"=1, "error in"=w263, "master data"="" ("Element 1"), "queue in"=w267) -> ("error out"=w266:errorcluster)  [unwired: 5 in, 1 out]
      }
      frame "<----------手动部分------------->" {
        w269 = u16 1 items=["HPRI"=1, "LPRI"=0] ("priority")
        # "//读取配置文件"
        n108 = call "Enqueue Element Array.vi"("priority"=w269, "queue index"=1, "error in"=w271, "master data"="" ("Element 1"), "queue in"=w275) -> ("error out"=w274:errorcluster)  [unwired: 5 in, 1 out]
      }
      frame "参数设置保存" {
        w277 = u16 1 items=["HPRI"=1, "LPRI"=0] ("priority")
        n109 = call "Enqueue Element Array.vi"("priority"=w277, "queue index"=1, "error in"=w279, "master data"="" ("Element 1"), "queue in"=w283) -> ("error out"=w282:errorcluster)  [unwired: 5 in, 1 out]
      }
      frame "<--------------手动结束---------------->" {
        w285 = u16 1 items=["HPRI"=1, "LPRI"=0] ("priority")
        # "//读取配置文件"
        n110 = call "Enqueue Element Array.vi"("priority"=w285, "queue index"=1, "error in"=w287, "master data"="" ("Element 1"), "queue in"=w291) -> ("error out"=w290:errorcluster)  [unwired: 5 in, 1 out]
      }
      frame "*Emergency alarm" {
        w300 = u16 1 items=["HPRI"=1, "LPRI"=0] ("priority")
        w301 = u16 1 items=["HPRI"=1, "LPRI"=0] ("priority")
        # "发出处理急停信号的命令"
        # "发出处理急停信号的命令"
        n111 = call "Enqueue Element Array.vi"("priority"=w300, "queue index"=0, "error in"=w294, "master data"="" ("Element 1"), "queue in"=w297) -> ("error out"=w295:errorcluster, "queue out"=w296:T12)  [unwired: 5 in]
        n112 = call "SetTestInfoIndex.vi"("test info index"=13) -> ()
        n113 = call "Enqueue Element Array.vi"("priority"=w301, "queue index"=1, "error in"=w295, "master data"="" ("Element 1"), "queue in"=w296) -> ("error out"=w305:errorcluster)  [unwired: 5 in, 1 out]
      }
    }
    n114 = Wait (ms)(milliseconds to wait=w131) -> ()  [unwired: 1 out]
  }
  n115 = call "Release Queue Array.vi"("error in"=w12, "queue in"=w10) -> ("error out"=w11:errorcluster)  [unwired: 2 in, 3 out]
  n116 = call "Release Queue Array.vi"("error in"=w15, "queue in"=w10) -> ("error out"=w18:errorcluster)  [unwired: 2 in, 3 out]
  n117 = call "MergeErrors.vi"("error in 3 (no error)"=w11, "error in 4 (no error)"=w18) -> ("error out"=w17:errorcluster)  [unwired: 6 in]
  n118 = call "ExitAppMode.vi"("error in (no error)"=w17) -> ("error out"=w16:errorcluster)  [unwired: 10 in]
  n119 = call <vilib>:"Clear Errors.vi"("error in (no error)"=w16) -> ()  [unwired: 5 in, 2 out]
  n120 = disable-structure shown="禁用" {
    disable-tunnel: "Search Direction (Contour Analysis 1)" -> [w315 _]
    disable-tunnel: "Contour Selection (Contour Analysis 1)" -> [w314 _]
    disable-tunnel: "Curve Connection (Contour Analysis 1)" -> [w313 _]
    disable-tunnel: "Curve Extraction 2 (Contour Analysis 1)" -> [w312 _]
    disable-tunnel: "Smoothing Kernel (Contour Analysis 1)" -> [w311 _]
    disable-tunnel: "Kernel Width (Contour Analysis 1)" -> [w310 _]
    disable-tunnel: "Template File Path (Contour Analysis 1)" -> [w309 _]
    disable-tunnel: "Match Mode (Contour Analysis 1)" -> [w308 _]
    disable-tunnel: "Curve Extraction (Contour Analysis 1)" -> [w307 _]
    frame Disabled {
      n121 = call "正面垫片处理方式2"("Curve Extraction (Contour Analysis 1)"=w307, "Search Direction (Contour Analysis 1)"=w315, "Contour Selection (Contour Analysis 1)"=w314, "Curve Connection (Contour Analysis 1)"=w313, "Kernel Width (Contour Analysis 1)"=w310, "Curve Extraction 2 (Contour Analysis 1)"=w312, "Template File Path (Contour Analysis 1)"=w309, "Match Mode (Contour Analysis 1)"=w308, "Smoothing Kernel (Contour Analysis 1)"=w311) -> ()  [unwired: 11 in, 8 out]
    }
    frame Enabled {
    }
  }
